vi "HexToBooleanArray.vi"() -> ()   [LabVIEW 2018]
panel:
  out "appended array":bool[](array[boolean])
  in  "String":string="8300000000008002"
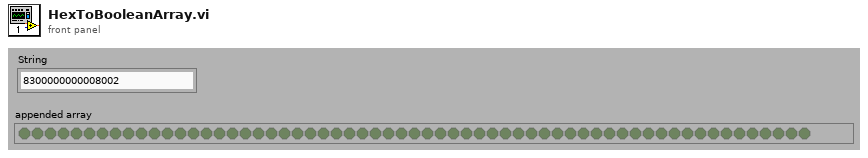
[diagram p1: front panel]
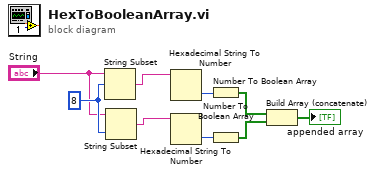
[diagram p0: block diagram]
diagram:
  w9 = 8 ("length (rest)")
  n1 = String Subset(string="String", offset (0)=w9) -> (substring=w8:string)  [unwired: 1 in]
  n2 = String Subset(string="String", length (rest)=w9) -> (substring=w7:string)  [unwired: 1 in]
  n3 = Hexadecimal String To Number(string=w8) -> (number=w6:u32)  [unwired: 2 in, 1 out]
  n4 = Hexadecimal String To Number(string=w7) -> (number=w5:u32)  [unwired: 2 in, 1 out]
  n5 = Number To Boolean Array(number=w6) -> (Boolean array=w4:bool[])
  n6 = Number To Boolean Array(number=w5) -> (Boolean array=w3:bool[])
  n7 = Build Array (concatenate)(w4, w3) -> (→"appended array":bool[])
